vi "SimpleDOwf.vi"(1 "size(s)":i32, 2 "Digital DC (%)":dbl, 3 "Digital time offset":dbl, 4 "Sampling frequency (Hz)":dbl, 5 "Digital Freq (Hz)":dbl, 6 "Digital phase (s)":dbl) -> (0 "digital waveform":digitalwaveform(waveform))   [LabVIEW 2015]
uses:
  <vilib>/Waveform/WDTOps.llb/WDT Append Waveforms DBL.vi
  <vilib>/Waveform/WDTOps.llb/WDT Get Waveform Subset DBL.vi
  <vilib>/Waveform/DWDTOps.llb/DWDT Analog to Digital.vi
  <vilib>/measure/NI_MABase.lvlib
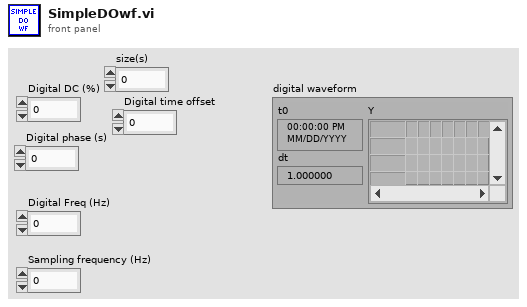
[diagram p1: front panel]
types:
  T1 = cluster{"Sampling frequency (Hz)":dbl, "size(s)":i32}
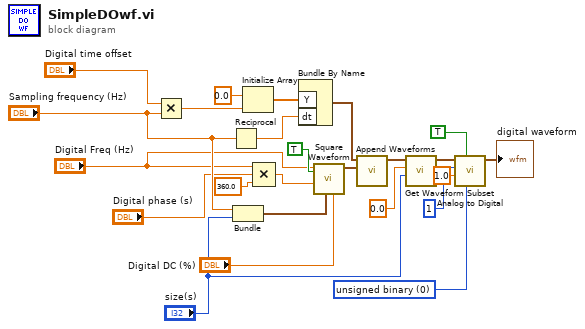
[diagram p0: block diagram]
diagram:
  w23 = u16 0 items=["unsigned binary", "offset binary", "2's complement"] ("data format (offset binary)")
  n1 = Multiply(x="Digital time offset", y="Sampling frequency (Hz)") -> (x*y=w17:dbl)
  n2 = Reciprocal(x="Sampling frequency (Hz)") -> (1/x=w19:dbl)
  n3 = Bundle("Sampling frequency (Hz)"="Sampling frequency (Hz)", "size(s)"="size(s)") -> (w21:T1)  [unwired: 1 in]
  n4 = Initialize Array(0.0 ("element"), w17) -> (w16:dbl[])
  n5 = Compound Arithmetic op=MULTIPLY("Digital Freq (Hz)", "Digital phase (s)", 360.0 ("value")) -> (w4:dbl)
  n6 = Bundle By Name("Y"=w16, "dt"=w19) -> (w14:waveform(dbl))  [unwired: 1 in]
  n7 = call <vilib>:"Square Waveform.vi"("duty cycle (%)"="Digital DC (%)", "sampling info"=w21, "reset signal"=TRUE, "phase"=w4, "frequency"="Digital Freq (Hz)") -> ("signal out"=w11:waveform(dbl))  [unwired: 5 in, 1 out]
  n8 = call-poly <vilib>:"Append Waveforms.vi"("waveform B"=w11, "waveform A"=w14) -> ("waveform out"=w13:waveform(dbl))  [unwired: 8 in, 1 out]
  n9 = call-poly <vilib>:"Get Waveform Subset.vi"("duration"="size(s)", "start samples/time"=0.0, "waveform in"=w13) -> ("waveform out"=w10:waveform(dbl))  [unwired: 3 in, 3 out]
  n10 = call-poly <vilib>:"Analog to Digital.vi"("data format (offset binary)"=w23, "compress digital (T)"=TRUE, "full-scale range (pk-pk)"=1.0, "resolution (16 bit)"=1, "analog waveform"=w10) -> ("digital waveform"=→"digital waveform":digitalwaveform)  [unwired: 3 in, 3 out]
